vi "Open Source Distribution.vi"(7 "TargetItem Refnum":refnum<vi>, 8 "error in (no error)":errorcluster, 10 "Build specification name":string, 11 "Project Refnum":refnum<vi>) -> (0 "error out":errorcluster, 3 "SDIST out":refnum<class "NI_AB_API_SDIST.lvclass">)   [LabVIEW 2020, in "NI_AB_API_SDIST.lvclass"]
uses:
  <vilib>/AppBuilder/AB_API/SDIST/NI_AB_API_SDIST.lvclass
  e:/builds/penguin/labview/branches/2020/dev/dist/vi.lib/AppBuilder/AB_API/Build/NI_AB_API_Build.lvclass
  <vilib>/AppBuilder/AB_API/common/AB_API Build Object Type.ctl
  <vilib>/AppBuilder/AB_Classes/Build/AB_Build.lvclass
  <vilib>/AppBuilder/AB_API/Build/NI_AB_API_Build.lvclass
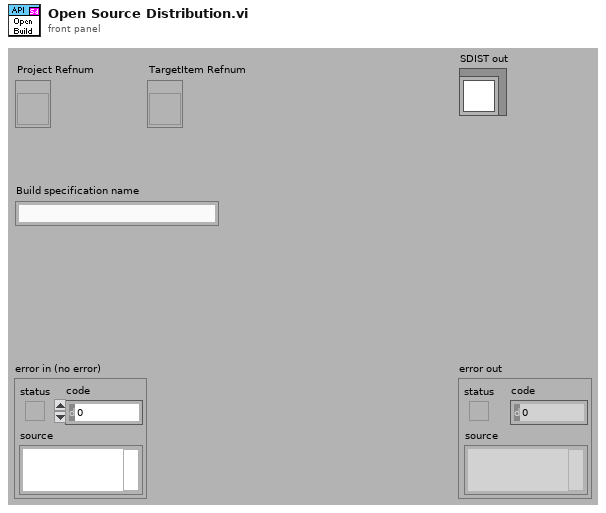
[diagram p1: front panel]
types:
  T1 = typedef "AB_API Build Object Type.ctl" = enum16{"Source Distribution", "DLL", "EXE", "Installer", "Zip File", "RESTful WS", "RTEXE", "Packed Library", "C Generation ", ".NET Interop Assembly"}
  T2 = typedef "ItemRef.ctl" = u64
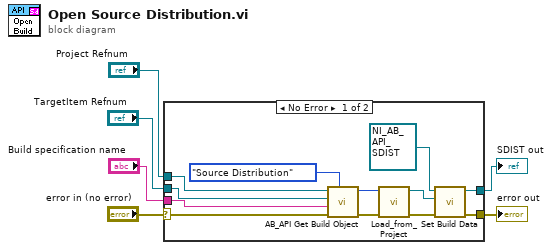
[diagram p0: block diagram]
diagram:
  n1 = case shown="No Error" "error in (no error)" {
    selector: "error in (no error)" -> [w14 w19]
    tunnel: [w11 w19] -> w5
    tunnel: [w10 _] -> w4
    tunnel: "Project Refnum" -> [w18 _]
    tunnel: "TargetItem Refnum" -> [w17 _]
    tunnel: "Build specification name" -> [w16 _]
    frame No Error {
      n2 = call <vilib>:"AB_API Get Build Object.vi"("Build object type"=AB_API_Build_Object_Type."Source Distribution", "error in (no error)"=w14, "Build spec name"=w16, "TargetItem Refnum"=w17, "Project Refnum"=w18) -> ("error out"=w12:errorcluster, "Build Object"=w13:T2)  [unwired: 5 in]
      n3 = call <vilib>:"Load_from_Project.vi"("error in (no error)"=w12, "Object"=w13) -> ("error out"=w8:errorcluster, "Build out"=w7:refnum<class "AB_Build.lvclass">)  [unwired: 8 in]
      n4 = call <vilib>:"Set Build Data.vi"("error in (no error)"=w8, "AB_Build.lvclass"=w7, "NI_AB_API_Build in"=refnum<class "NI_AB_API_SDIST.lvclass"> refnum ("NI_AB_API_SDIST.lvclass")) -> ("error out"=w11:errorcluster, "NI_AB_API_Build out"=w10:refnum<class "NI_AB_API_SDIST.lvclass">)  [unwired: 7 in]
    }
    frame Error {
    }
  }
  "error out" <- w5
  "SDIST out" <- w4
